vi "Queue Driver-Sender.vi"(0 "States[]":string[](array[string]), 5 "State":string, 7 "Data":variant, 9 "Queue Name":string, 11 "Error In":errorcluster, 13 "Queue Operation":T2) -> (4 "Dequeue Element":T1, 15 "Error Out":errorcluster)   [LabVIEW 2023]
doc: "The VI performs the queue operations. The operations include create, enqueue, dequeue, flush and closes the queue."
uses:
  Controls/Queue Operation.ctl
  Controls/Queue Element.ctl
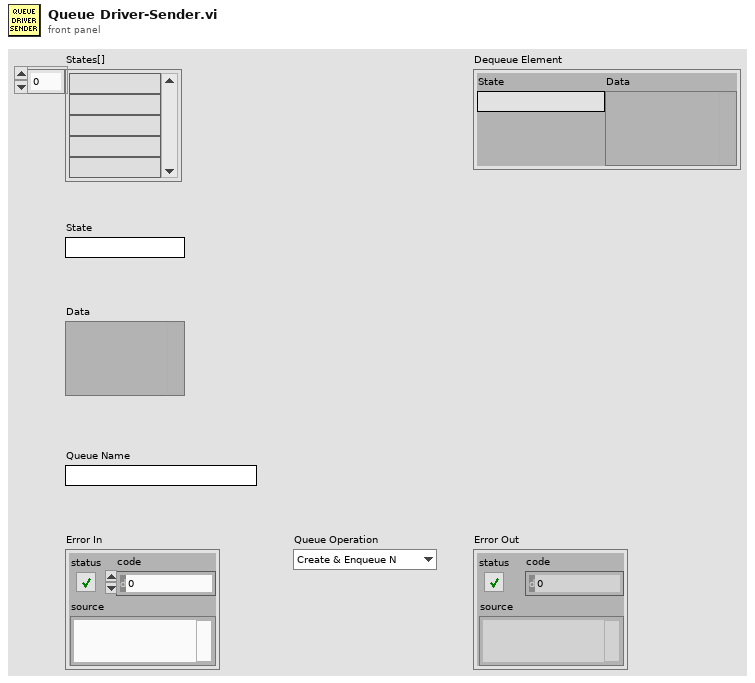
[diagram p1: front panel]
types:
  T1 = typedef "Queue Element.ctl" = cluster{"State":string, "Data":variant}
  T2 = typedef "Queue Operation.ctl" = enum16{"Create & Enqueue N", "Enqueue N", "Dequeue", "Enstack N", "Flush", "Release"}
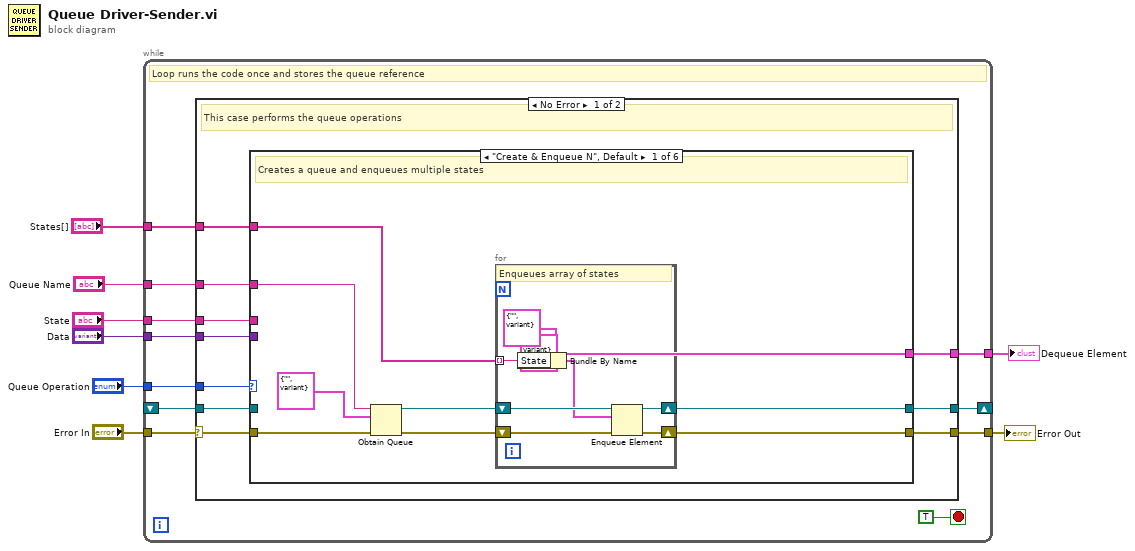
[diagram p0: block diagram]
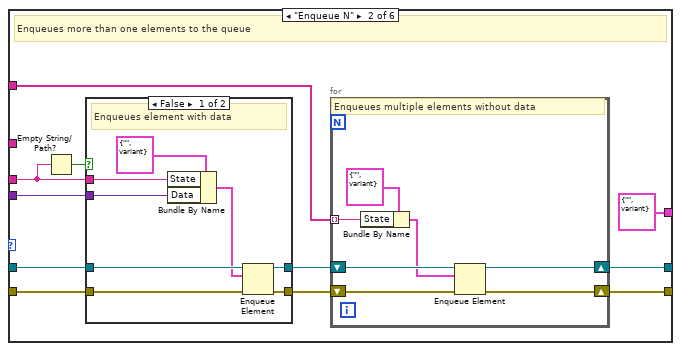
[diagram p2: hidden frame]
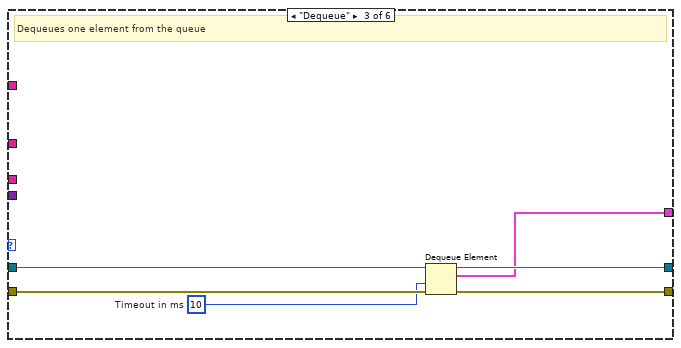
[diagram p4: hidden frame]
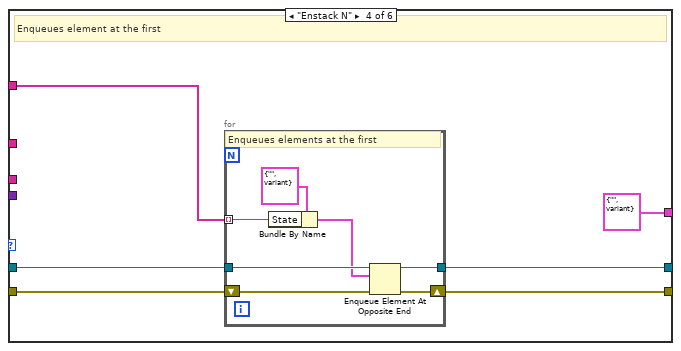
[diagram p5: hidden frame]
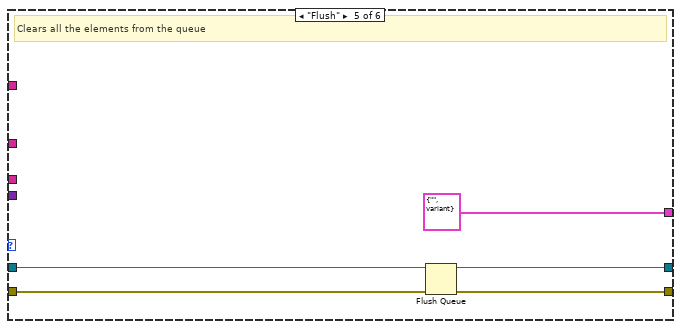
[diagram p6: hidden frame]
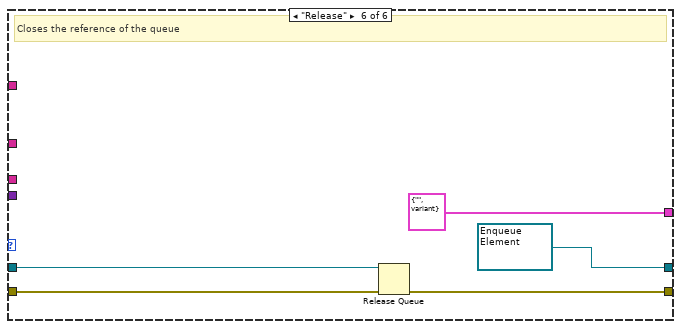
[diagram p7: hidden frame]
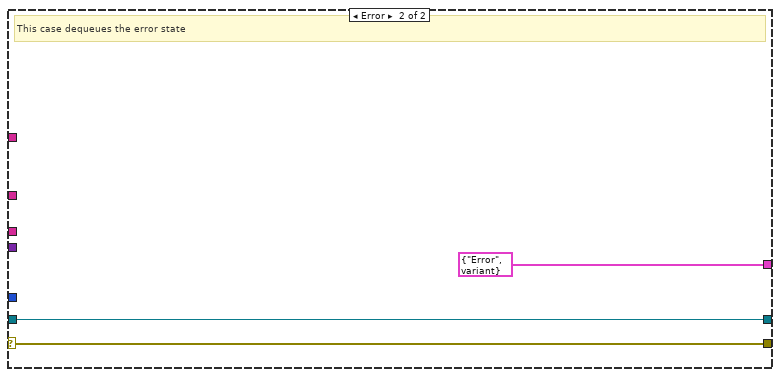
[diagram p8: hidden frame]
diagram:
  n1 = while {
    tunnel: "Error In" -> [w19]
    tunnel: "Queue Operation" -> [w18]
    tunnel: "Queue Name" -> [w17]
    shift-right: [w16] -> _
    shift-left: _ -> [w15]
    tunnel: [w14] -> w5
    tunnel: [w12] -> w4
    tunnel: "Data" -> [w11]
    tunnel: "State" -> [w10]
    tunnel: "States[]" -> [w9]
    stop <- TRUE stop-if-true
    # "Loop runs the code once and stores the queue reference"
    n2 = case shown="No Error" w19 {
      selector: w19 -> [w29 w104]
      tunnel: w18 -> [w28 _]
      tunnel: w17 -> [w27 _]
      tunnel: [w26 w105] -> w16
      tunnel: w15 -> [w25 w105]
      tunnel: [w24 w104] -> w14
      tunnel: [w23 T1 {"State"="Error", "Data"=variant} ("Dequeue Element")] -> w12
      tunnel: w11 -> [w22 _]
      tunnel: w10 -> [w21 _]
      tunnel: w9 -> [w20 _]
      frame No Error {
        # "This case performs the queue operations"
        n3 = case shown="\"Create & Enqueue N\", Default" w28 {
          tunnel: [w32 w55 w78 w84 w96 w101] -> w24
          tunnel: w29 -> [w38 w56 w79 w85 w97 w102]
          tunnel: w27 -> [w37 _ _ _ _ _]
          tunnel: [w33 w54 w77 w82 w94 refnum<queue> refnum ("queue out")] -> w26
          tunnel: w25 -> [_ w50 w76 w83 w95 w100]
          tunnel: [T1 {"State"="", "Data"=variant} ("Dequeue Element") T1 {"State"="", "Data"=variant} ("Dequeue Element") w74 T1 {"State"="", "Data"=variant} ("Dequeue Element") T1 {"State"="", "Data"=variant} ("Dequeue Element") T1 {"State"="", "Data"=variant} ("Dequeue Element")] -> w23
          tunnel: w22 -> [_ w48 _ _ _ _]
          tunnel: w21 -> [_ w47 _ _ _ _]
          tunnel: w20 -> [w30 w52 _ w81 _ _]
          frame "Create & Enqueue N", Default {
            # "Creates a queue and enqueues multiple states"
            n4 = Obtain Queue(name (unnamed)=w37, element data type=T1 {"State"="", "Data"=variant} ("Dequeue Element"), error in (no error)=w38) -> (queue out=w34:refnum<queue>, error out=w31:errorcluster)  [unwired: 2 in, 1 out]
            n5 = for {
              shift-right: [w44] -> w32
              shift-left: w31 -> [w45]
              tunnel: w30 -> [w39] mode=indexing
              shift-right: [w42] -> w33
              shift-left: w34 -> [w43]
              # "Enqueues array of states"
              n6 = Bundle By Name(cluster=T1 {"State"="", "Data"=variant} ("Dequeue Element"), "State"=w39) -> (w41:T1)
              n7 = Enqueue Element(queue=w43, element=w41, error in (no error)=w45) -> (queue out=w42:refnum<queue>, error out=w44:errorcluster)  [unwired: 1 in, 1 out]
            }
          }
          frame "Enqueue N" {
            # "Enqueues more than one elements to the queue"
            n8 = Empty String/Path?(string/path=w47) -> (empty?=w46:bool)
            n9 = case shown="False" w46 {
              tunnel: w56 -> [w64 w65]
              tunnel: [w63 w65] -> w51
              tunnel: w50 -> [w62 w66]
              tunnel: [w61 w66] -> w49
              tunnel: w47 -> [w60 _]
              tunnel: w48 -> [w57 _]
              frame False {
                # "Enqueues element with data"
                n10 = Bundle By Name(cluster=T1 {"State"="", "Data"=variant} ("Dequeue Element"), "State"=w60, "Data"=w57) -> (w58:T1)
                n11 = Enqueue Element(queue=w62, element=w58, error in (no error)=w64) -> (queue out=w61:refnum<queue>, error out=w63:errorcluster)  [unwired: 1 in, 1 out]
              }
              frame True {
              }
            }
            n12 = for {
              shift-right: [w72] -> w55
              shift-left: w51 -> [w73]
              tunnel: w52 -> [w67] mode=indexing
              shift-right: [w70] -> w54
              shift-left: w49 -> [w71]
              # "Enqueues multiple elements without data"
              n13 = Bundle By Name(cluster=T1 {"State"="", "Data"=variant} ("Dequeue Element"), "State"=w67) -> (w69:T1)
              n14 = Enqueue Element(queue=w71, element=w69, error in (no error)=w73) -> (queue out=w70:refnum<queue>, error out=w72:errorcluster)  [unwired: 1 in, 1 out]
            }
          }
          frame "Dequeue" {
            w75 = 10  # Timeout in ms
            # "Dequeues one element from the queue"
            n15 = Dequeue Element(queue=w76, timeout in ms (-1)=w75, error in (no error)=w79) -> (queue out=w77:refnum<queue>, element=w74:T1, error out=w78:errorcluster)  [unwired: 1 out]
          }
          frame "Enstack N" {
            # "Enqueues element at the first"
            n16 = for {
              tunnel: w83 -> [w90]
              tunnel: [w89] -> w82
              shift-right: [w91] -> w84
              shift-left: w85 -> [w92]
              tunnel: w81 -> [w86] mode=indexing
              # "Enqueues elements at the first"
              n17 = Bundle By Name(cluster=T1 {"State"="", "Data"=variant} ("Enqueue Element"), "State"=w86) -> (w88:T1)
              n18 = Enqueue Element At Opposite End(queue=w90, element=w88, error in (no error)=w92) -> (queue out=w89:refnum<queue>, error out=w91:errorcluster)  [unwired: 1 in, 1 out]
            }
          }
          frame "Flush" {
            # "Clears all the elements from the queue"
            n19 = Flush Queue(queue=w95, error in (no error)=w97) -> (queue out=w94:refnum<queue>, error out=w96:errorcluster)  [unwired: 1 out]
          }
          frame "Release" {
            # "Closes the reference of the queue"
            n20 = Release Queue(queue=w100, error in (no error)=w102) -> (error out=w101:errorcluster)  [unwired: 1 in, 2 out]
          }
        }
      }
      frame Error {
        # "This case dequeues the error state"
      }
    }
  }
  "Error Out" <- w5
  "Dequeue Element" <- w4
